vi "GSI-HVSwitch2.read temp amp.vi"(0 "i ref in":refnum<vi>, 3 "ms timeout (10000)":i32=10000, 5 "error in (no error)":errorcluster) -> (14 "i ref out":refnum<vi>, 16 "ActTempAmp":dbl format="%.2f", 17 "timed out":bool, 19 "error out":errorcluster)   [LabVIEW 2014, in "GSI-HVSwitch2.lvlib"]
doc: "Reads the temperature of the amplifier chip"
uses:
  GSI-HVSwitch2.lvlib
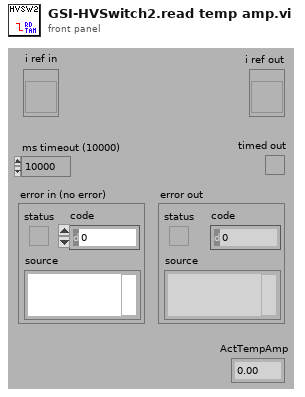
[diagram p1: front panel]
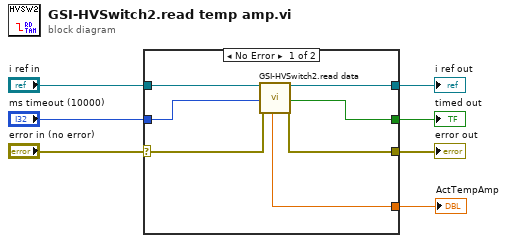
[diagram p0: block diagram]
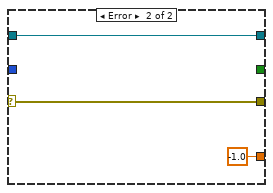
[diagram p2: hidden frame]
diagram:
  n1 = case shown="No Error" "error in (no error)" {
    selector: "error in (no error)" -> [w8 w16]
    tunnel: "i ref in" -> [w14 w17]
    tunnel: "ms timeout (10000)" -> [w13 _]
    tunnel: [w12 _] -> w5
    tunnel: [w11 w17] -> w4
    tunnel: [w10 w16] -> w3
    tunnel: [w9 -1.0 ("ActTempAmp")] -> w2
    frame No Error {
      n2 = call "GSI-HVSwitch2.read data.vi"("i ref in"=w14, "ms timeout (10000)"=w13, "error in (no error)"=w8) -> ("ActTempAmp"=w9:dbl, "i ref out"=w11:refnum<vi>, "timed out"=w12:bool, "error out"=w10:errorcluster)  [unwired: 10 in, 3 out]
    }
    frame Error {
    }
  }
  "error out" <- w3
  "i ref out" <- w4
  "timed out" <- w5
  "ActTempAmp" <- w2
